vi "Interpolate 2D Scattered_Wn.vi"(0 "X(Tri) In":dbl[][](array[numeric]), 5 "Y(Tri) In":dbl[][](array[numeric]), 7 "Z(Tri) In":dbl[][](array[numeric]), 9 "gx in":dbl[][](array[numeric]), 11 "gy in":dbl[][](array[numeric]), 12 "Length":dbl[][](array[numeric])) -> (4 "X(Tri) Out":dbl[][](array[numeric]), 6 "Y(Tri) Out":dbl[][](array[numeric]), 8 "Z(Tri) Out":dbl[][](array[numeric]), 10 "gx out":dbl[][](array[numeric]), 14 "Wn":dbl[][](array[numeric]), 15 "gy out":dbl[][](array[numeric]))   [LabVIEW 2017, in "NI_AAL_Interpolation.lvlib"]
uses:
  <vilib>/gmath/NI_AAL_Interpolation.lvlib
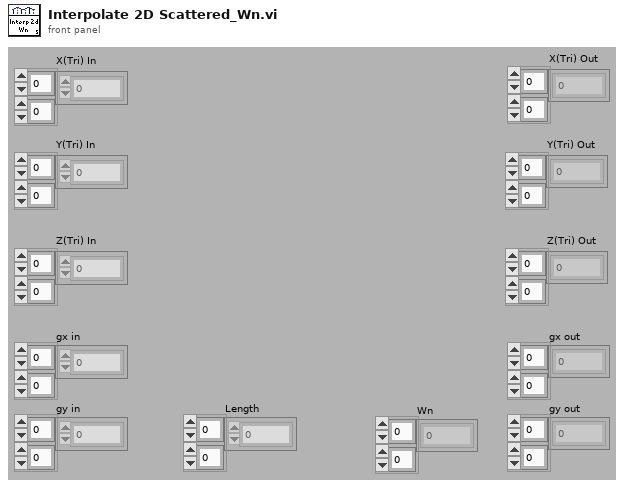
[diagram p1: front panel]
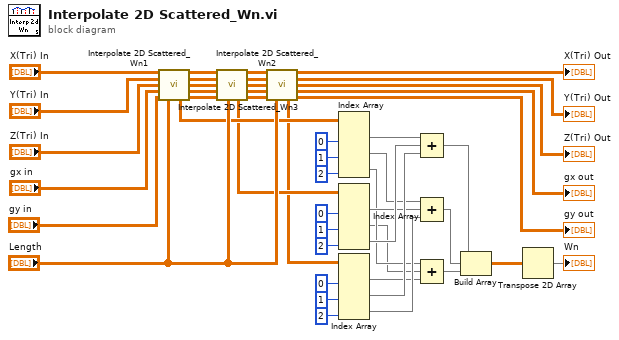
[diagram p0: block diagram]
diagram:
  n1 = call <vilib>:"Interpolate 2D Scattered_Wn1.vi"("X(Tri) In"="X(Tri) In", "Y(Tri) In"="Y(Tri) In", "Z(Tri) In"="Z(Tri) In", "gx in"="gx in", "gy in"="gy in", "Length"="Length") -> ("X(Tri) Out"=w19:dbl[][], "Y(Tri) Out"=w18:dbl[][], "Z(Tri) Out"=w17:dbl[][], "gx out"=w16:dbl[][], "Wn 1"=w8:dbl[][], "gy out"=w15:dbl[][])  [unwired: 4 in]
  n2 = call <vilib>:"Interpolate 2D Scattered_Wn2.vi"("X(Tri) In"=w19, "Y(Tri) In"=w18, "Z(Tri) In"=w17, "gx in"=w16, "gy in"=w15, "Length"="Length") -> ("X(Tri) Out"=w14:dbl[][], "Y(Tri) Out"=w13:dbl[][], "Z(Tri) Out"=w12:dbl[][], "gx out"=w11:dbl[][], "Wn 2"=w7:dbl[][], "gy out"=w10:dbl[][])  [unwired: 4 in]
  n3 = call <vilib>:"Interpolate 2D Scattered_Wn3.vi"("X(Tri) In"=w14, "Y(Tri) In"=w13, "Z(Tri) In"=w12, "gx in"=w11, "gy in"=w10, "Length"="Length") -> ("X(Tri) Out"=→"X(Tri) Out":dbl[][], "Y(Tri) Out"=→"Y(Tri) Out":dbl[][], "Z(Tri) Out"=→"Z(Tri) Out":dbl[][], "gx out"=→"gx out":dbl[][], "Wn 3"=w6:dbl[][], "gy out"=→"gy out":dbl[][])  [unwired: 4 in]
  n4 = Index Array(array=w8, index (col) #1=0 ("disabled index (col)"), index (col) #2=1 ("index (col)"), index (col) #3=2 ("index (col)")) -> (element #1=w38:dbl[], element #2=w34:dbl[], element #3=w32:dbl[])  [unwired: 3 in]
  n5 = Index Array(array=w7, index (col) #1=0 ("disabled index (col)"), index (col) #2=1 ("index (col)"), index (col) #3=2 ("index (col)")) -> (element #1=w35:dbl[], element #2=w31:dbl[], element #3=w37:dbl[])  [unwired: 3 in]
  n6 = Index Array(array=w6, index (col) #1=0 ("disabled index (col)"), index (col) #2=1 ("index (col)"), index (col) #3=2 ("index (col)")) -> (element #1=w30:dbl[], element #2=w36:dbl[], element #3=w33:dbl[])  [unwired: 3 in]
  n7 = Compound Arithmetic op=ADD(w38, w37, w36) -> (w29:dbl[])
  n8 = Compound Arithmetic op=ADD(w34, w35, w33) -> (w28:dbl[])
  n9 = Compound Arithmetic op=ADD(w32, w31, w30) -> (w27:dbl[])
  n10 = Build Array(w29, w28, w27) -> (w26:dbl[][])
  n11 = Transpose 2D Array(2D array=w26) -> (transposed array=→"Wn":dbl[][])
